vi "Write Voltage Power Supply.vi"(9 "Voltage":dbl(knob) min=0.0 max=5.0, 10 "Channel":enum16{"Positive", "Negative"}(ring), 11 "ADALM2000 Handler":u64 caption="Instrument Handle Out") -> (3 "ADALM2000 Handler 2":u64 caption="Instrument Handle Out")   [LabVIEW 2022 SP3]
uses:
  libm2k_lv.dll
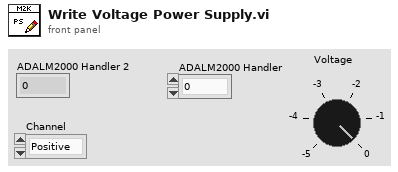
[diagram p1: front panel]
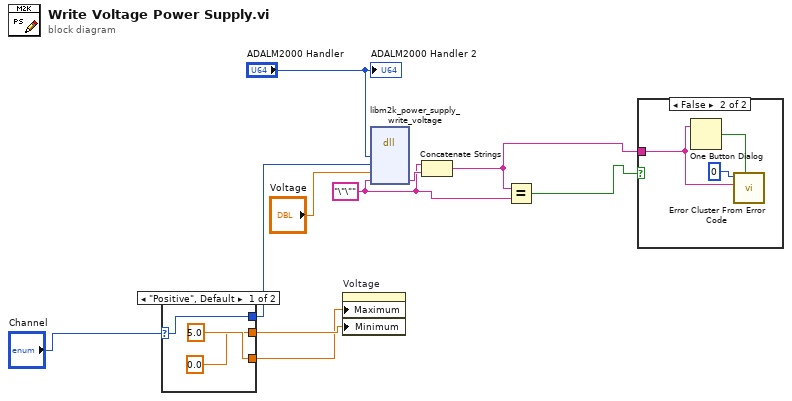
[diagram p0: block diagram]
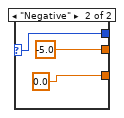
[diagram p2: hidden frame]
diagram:
  w8 = "\"\""
  n1 = case shown="\"Positive\", Default" "Channel" {
    selector: "Channel" -> [w11 w14]
    tunnel: [0.0 -5.0] -> w4
    tunnel: [5.0 0.0] -> w3
    tunnel: [w11 w14] -> w1
    frame "Positive", Default {
    }
    frame "Negative" {
    }
  }
  n2 = property on="Voltage" class="Knob (strict)"("Maximum"=w3, "Minimum"=w4) -> ()  [unwired: 2 in, 2 out]
  n3 = dll-call lib="libm2k_lv.*" fn="libm2k_power_supply_write_voltage"("instance"="ADALM2000 Handler", "chnIdx"=w1, "value"="Voltage", "err"=w8) -> ("err"=w10:string)  [unwired: 7 in, 2 out]
  n4 = Concatenate Strings(w8, w10) -> (w6:string)
  n5 = Equal?(x=w6, y=w8) -> (x = y?=w7:bool)
  n6 = case shown="False" w7 {
    tunnel: w6 -> [_ w17]
    frame True {
    }
    frame False {
      n7 = One Button Dialog(message=w17) -> (true=w19:bool)  [unwired: 1 in]
      n8 = call <vilib>:"Error Cluster From Error Code.vi"("show call chain? (False)"=w19, "error message (\"\")"=w17, "error code (0)"=0) -> ()  [unwired: 6 in, 1 out]
    }
  }
  "ADALM2000 Handler 2" <- "ADALM2000 Handler"
